vi "Start.vi"(8 "error in (no error)":errorcluster, 10 "Message in":refnum<class "StartMessage.lvclass">, 11 "AOTF in":refnum<class "AOTF.lvclass">) -> (0 "error out":errorcluster, 3 "AOTF out":refnum<class "AOTF.lvclass">)   [LabVIEW 2012, in "AOTF.lvclass"]
doc: "This member function is called when the statemachine in the run.vi receives an 'start' command. It relays the message to all observers of the component.\n\nOverride this member function in your derived class if you need additional start functionality (but don't forget to call the parent method)."
uses:
  AOTF.lvclass
  <vilib>/Distrio/Murmex/StartMessage/StartMessage.lvclass
  <vilib>/Distrio/Murmex/Murmex/Murmex.lvclass
panel:
  # "This member function is called when the statemachine in the run.vi receives an 'start' command. It relays the message to all observers of the component.\n\nOverride this member function in your derived class if you need additional start functionality (but don't forget to call the parent method)."
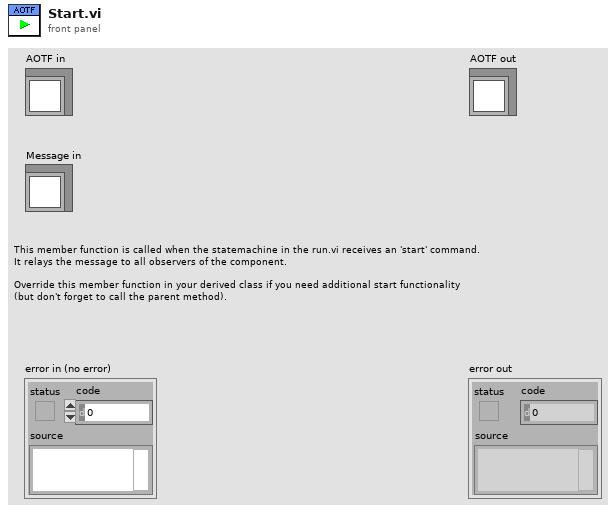
[diagram p1: front panel]
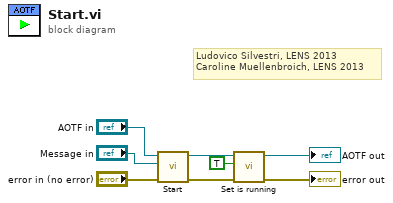
[diagram p0: block diagram]
diagram:
  # "Ludovico Silvestri, LENS 2013\nCaroline Muellenbroich, LENS 2013"
  n1 = call-parent "Start.vi"("error in (no error)"="error in (no error)", "Message in"="Message in", "Murmex in"="AOTF in") -> ("error out"=w5:errorcluster, "Murmex out"=w3:refnum<class "AOTF.lvclass">)  [unwired: 7 in]
  n2 = call-dynamic "Set is running.vi"("error in (no error)"=w5, "is running?"=TRUE, "AOTF in"=w3) -> ("error out"=→"error out":errorcluster, "AOTF out"=→"AOTF out":refnum<class "AOTF.lvclass">)  [unwired: 7 in]
